vi "Write Binary as Value.vi"(8 "error in (no error)":errorcluster, 9 "Binary":string, 10 "Tag":string, 11 "Var Bus in":refnum<class "Omni_Bus.lvclass">) -> (0 "error out":errorcluster, 3 "Var Bus out":refnum<class "Omni_Bus.lvclass">)   [LabVIEW 2021, in "Omni_Bus.lvclass"]
uses:
  Omni_Bus.lvclass
  <vilib>/TSA/Abstract Data Classes/Abs_Types/Value/Abs_Value.lvclass
  C:/Program Files (x86)/National Instruments/LabVIEW 2021/vi.lib/TSA/Abstract Data Classes/Abs_Types/Type/Abs_Type.lvclass
  <vilib>/TSA/Abstract Data Classes/Abs_Types/Type/Abs_Type.lvclass/Abs_Type.ctl
  Omni_Bus.lvclass/Omni_Bus.ctl
  <vilib>/Utility/error.llb/Clear Errors.vi
  Properties/Read Var Map.vi
  <vilib>/TSA/Abstract Data Classes/Abs_Types/Type/Properties/Read Tag.vi
  Check For Read Only Error.vi
  Incorrect Tag String Error.vi
  <vilib>/TSA/Abstract Data Classes/Abs_Types/Type/Abs_Type.lvclass
  C:/Program Files (x86)/National Instruments/LabVIEW 2021/vi.lib/TSA/Abstract Data Classes/Abs_Types/Value/Abs_Value.lvclass
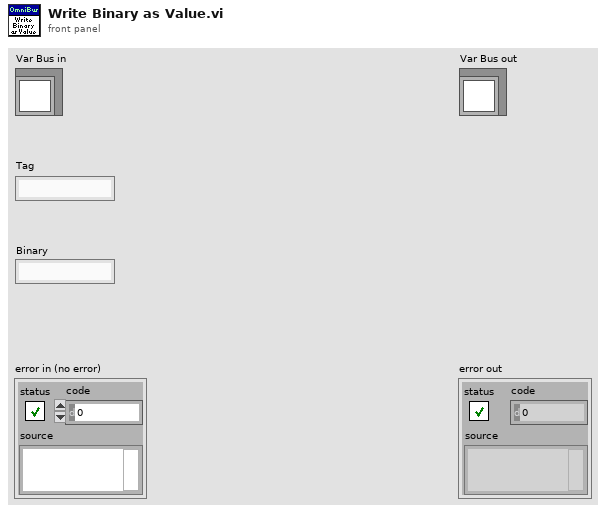
[diagram p1: front panel]
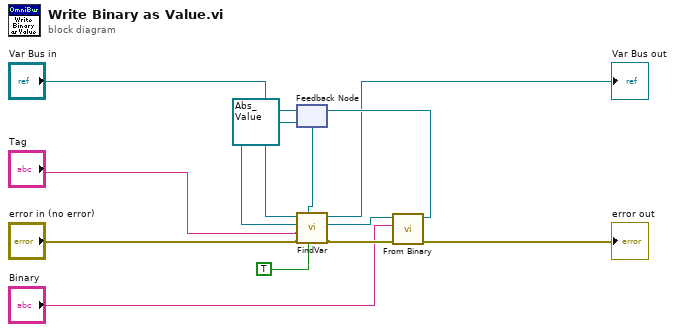
[diagram p0: block diagram]
diagram:
  w1 = refnum<class "Abs_Value.lvclass"> refnum ("Type out")
  n1 = feedback #1(w1) -> (w6:refnum<class "Abs_Value.lvclass">)
  n2 = call "FindVar.vi"("Write?"=TRUE, "Abs_Type"=w1, "error in (no error)"="error in (no error)", "Tag"="Tag", "Abs_Type Default"=w6, "Var Bus in"="Var Bus in") -> ("error out"=w10:errorcluster, "Abs_Type Found"=w9:refnum<class "Abs_Value.lvclass">, "Var Bus out"=→"Var Bus out":refnum<class "Omni_Bus.lvclass">)  [unwired: 2 in, 1 out]
  n3 = call-dynamic "From Binary.vi"("error in (no error)"=w10, "Binary"="Binary", "Type in"=w9) -> ("error out"=→"error out":errorcluster, "Type out"=w11:refnum<class "Abs_Value.lvclass">)  [unwired: 6 in, 1 out]
  n4 = feedback-in #1(w11) -> ()
